vi "MotorTest.vi"() -> ()   [LabVIEW 2014]
panel:
  in  "Desired Position":i32
  out "Position Out":i32
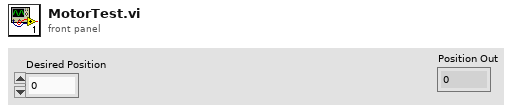
[diagram p1: front panel]
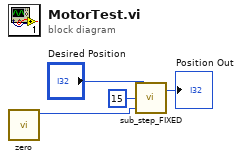
[diagram p0: block diagram]
diagram:
  n1 = call "zero.vi"() -> ("PositionOut"=w4:i32)  [unwired: 11 in]
  n2 = call "sub_step_FIXED.vi"("Current Position"=w4, "millisecond multiple"=u32 15, "Desired Position"="Desired Position") -> ("Position Out"=→"Position Out":i32)  [unwired: 1 in]
